vi "iow56_adc.vi"() -> ()   [LabVIEW 2011]
panel:
  out "Report 2":u8[](array[numeric]) format="%.0x"
  out "Volt AD0":dbl
  out "RAW AD01":i32
  out "Error":errorcluster caption="error"
  out "Report":u8[](array[numeric]) format="%.0x"
  in  "Stopp":bool
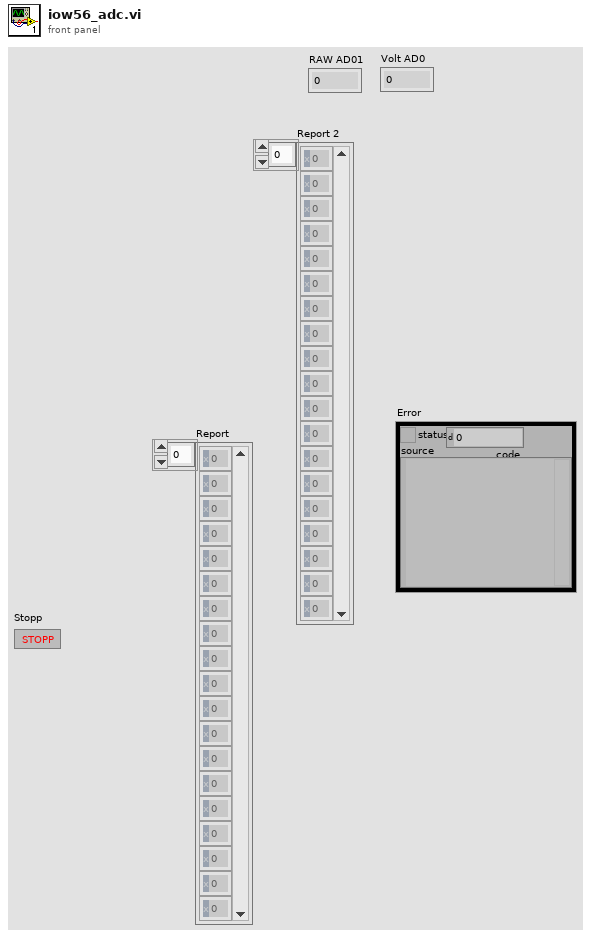
[diagram p1: front panel]
types:
  T1 = typedef "IOWarrior_Handle.ctl" = cluster{"Handle":u32, "Serial Number":string, "type of Warrior":T2, "Root Handle":bool, "Revision":u16}
  T2 = typedef "IOWarrior_Type.ctl" = enum16{"invalid", "IOW24", "IOW40", "IOW56", "IOPV1", "IOPV2"}
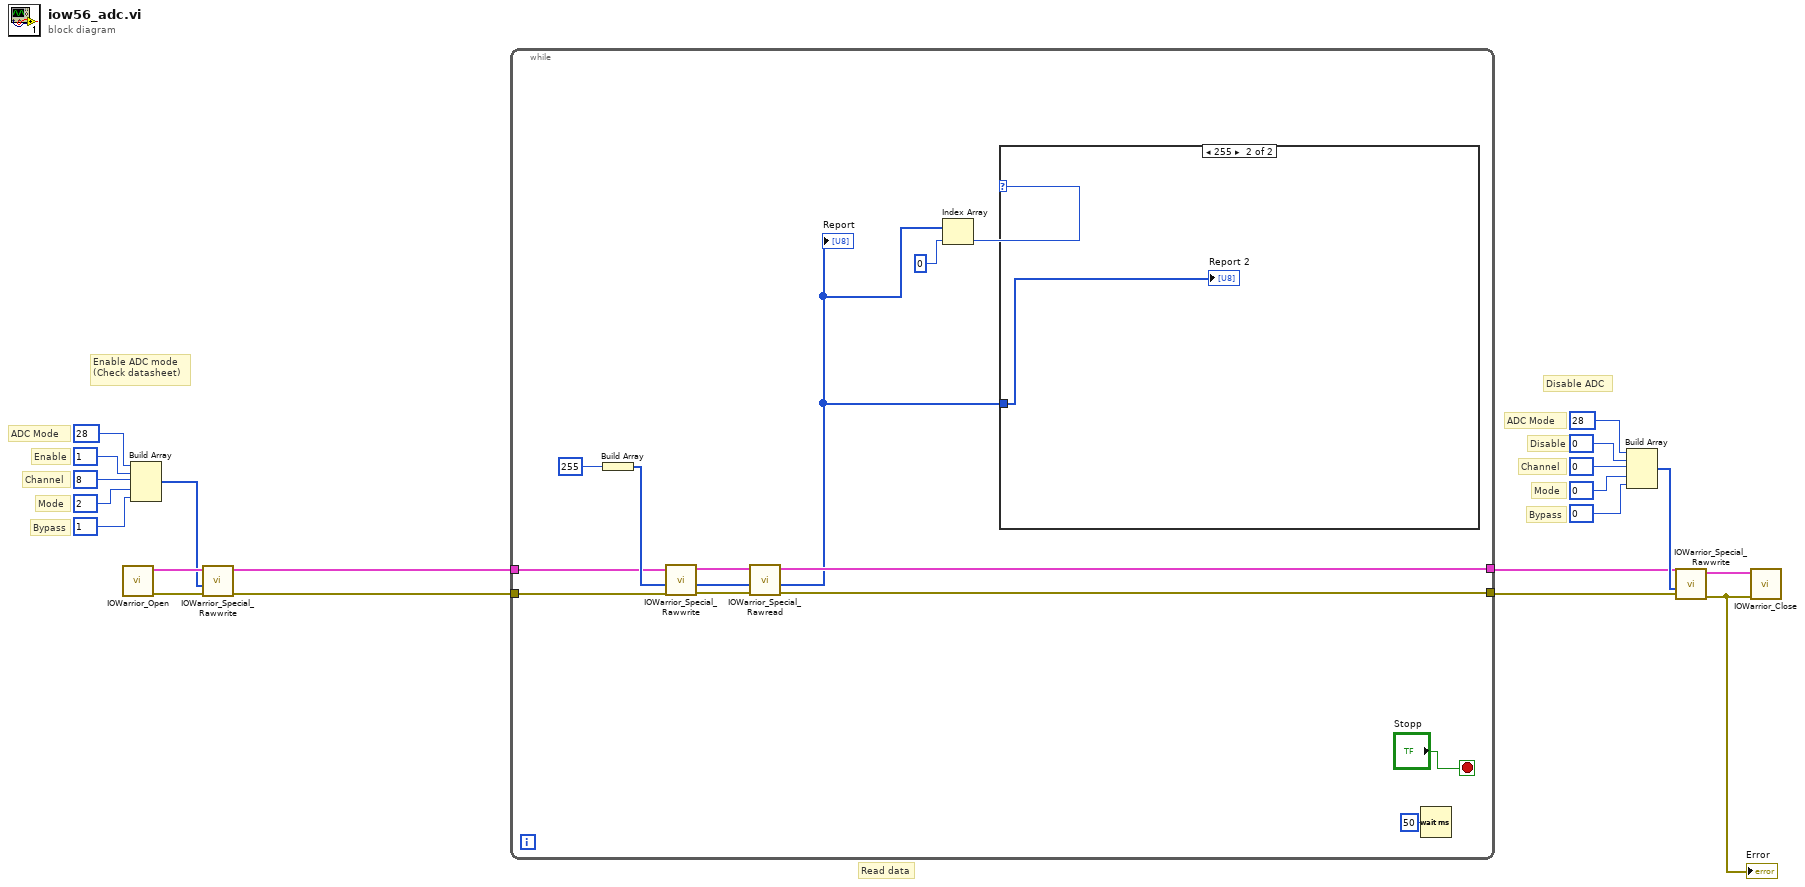
[diagram p0: block diagram]
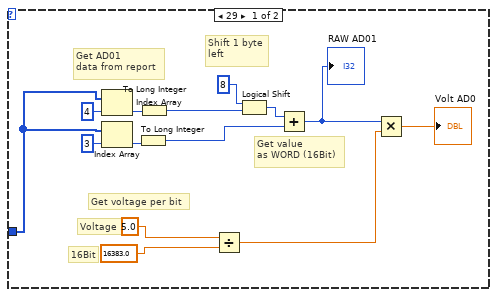
[diagram p2: hidden frame]
diagram:
  # "Disable ADC"
  # "Bypass"
  # "Mode"
  # "Channel"
  # "Disable"
  # "ADC Mode"
  # "Read data"
  # "Enable ADC mode\n(Check datasheet)"
  # "Bypass"
  # "Mode"
  # "Channel"
  # "Enable"
  # "ADC Mode"
  n1 = call "IOWarrior_Open.vi"() -> ("err out"=w14:errorcluster, "IOWarriorHandle"=w15:T1)  [unwired: 9 in, 1 out]
  n2 = Build Array(u8 28, u8 1, u8 8, u8 2, u8 1) -> (w13:u8[])
  n3 = call "IOWarrior_Special_Rawwrite.vi"("err in"=w14, "Array_in"=w13, "devHandle"=w15) -> ("err out"=w12:errorcluster, "devHandleout"=w1:T1)  [unwired: 6 in, 1 out]
  n4 = while {
    tunnel: w12 -> [w26]
    tunnel: [w31] -> w4
    tunnel: [w33] -> w3
    tunnel: w1 -> [w27]
    stop <- "Stopp" stop-if-true
    n5 = Build Array(u8 255) -> (w28:u8[])
    n6 = call "IOWarrior_Special_Rawwrite.vi"("err in"=w26, "Array_in"=w28, "devHandle"=w27) -> ("err out"=w24:errorcluster, "array_out"=w23:u8[], "devHandleout"=w25:T1)  [unwired: 6 in]
    n7 = call "IOWarrior_Special_Rawread.vi"("err in"=w24, "array"=w23, "devHandle"=w25) -> ("err out"=w33:errorcluster, "arrayout"=w21:u8[], "devHandleout"=w31:T1)  [unwired: 6 in]
    "Report" <- w21
    n8 = Index Array(array=w21, index=0) -> (element=w22:u8)
    n9 = case shown="255" w22 {
      tunnel: w21 -> [w35 w49]
      frame 29 {
        # "16Bit"
        # "Voltage"
        # "Get AD01\ndata from report"
        # "Get value\nas WORD (16Bit)"
        # "Get voltage per bit"
        # "Shift 1 byte\nleft"
        n10 = Index Array(array=w35, index=4) -> (element=w39:u8)
        n11 = Index Array(array=w35, index=3) -> (element=w37:u8)
        n12 = To Long Integer(number=w37) -> (32bit integer=w36:i32)
        n13 = To Long Integer(number=w39) -> (32bit integer=w38:i32)
        n14 = Divide(x=5.0, y=16383.0) -> (x/y=w41:dbl)
        n15 = Logical Shift(y=8, x=w38) -> (x << y=w46:i32)
        n16 = Add(x=w46, y=w36) -> (x+y=w45:i32)
        "RAW AD01" <- w45
        n17 = Multiply(x=w45, y=w41) -> (x*y=→"Volt AD0":dbl)
      }
      frame 255 {
        "Report 2" <- w49
      }
    }
    n18 = Wait (ms)(milliseconds to wait=50) -> ()  [unwired: 1 out]
  }
  n19 = Build Array(u8 28, u8 0, u8 0, u8 0, u8 0) -> (w5:u8[])
  n20 = call "IOWarrior_Special_Rawwrite.vi"("err in"=w3, "Array_in"=w5, "devHandle"=w4) -> ("err out"=w2:errorcluster, "devHandleout"=w11:T1)  [unwired: 6 in, 1 out]
  "Error" <- w2
  n21 = call "IOWarrior_Close.vi"("err in"=w2, "devHandle"=w11) -> ()  [unwired: 8 in, 2 out]
